vi "Module_ENG_SnakeProcessor.vi"(8 "error in (no error)":errorcluster, 9 "Module ID (-1: Do not Address)":i32=-1, 10 "Wait on Module(s) (\"\": none)":string) -> (0 "error out":errorcluster)   [LabVIEW 2019, in "Module_ENG_SnakeProcessor.lvclass"]
doc: "created using\nJSMA Module Template - ENGINE Class 0.2.1.12\nRob Humfeld - Jet Engineering\nCopyright (c) 2020, Jet Engineering"
uses:
  Module_ENG_SnakeProcessor.lvclass
  <userlib>/Jet Engineering/JET_QSM/Code/Private/JET_QSM - Add State to Front [String API].vi
  Private/Module_ENG_SnakeProcessor_jMsgTxList STYP.ctl
  Private/Module_ENG_SnakeProcessor_jMsgRxList STYP.ctl
  <userlib>/Jet Engineering/JET_QSM/Code/Private/JET_QSM_InvalidOption STYP.ctl
  <userlib>/Jet Engineering/JET_QSM/Code/Private/JET_QSM - Add State [String API].vi
  Private/Module_ENG_SnakeProcessor_EngineStatus STYP.ctl
  Private/Module_ENG_SnakeProcessor_LocalData STYP.ctl
  <userlib>/Jet Engineering/JSMA/Libraries/jMsg_CORE/jMsg_JSMA_ModuleOnline/jMsg_JSMA_ModuleOnline.lvclass
  <userlib>/Jet Engineering/JSMA/Libraries/jMsg_CORE/jMsg_JSMA_ApplicationShutdown/jMsg_JSMA_ApplicationShutdown.lvclass
  <userlib>/Jet Engineering/JSMA/Libraries/jModule Class/jModule.lvclass
  Shared/TCP/jMsgs/jMsg_TCPMessage_Receive/jMsg_TCPMessage_Receive.lvclass
  <userlib>/Jet Engineering/JSMA/Libraries/jMsg Class/jMsg.lvclass
  Shared/TCP/jMsgs/jMsg_TCPMessage_Send/jMsg_TCPMessage_Send.lvclass
  Shared/Board/Board.lvclass
  Shared/jMsgs/jMsg_SnakeProcessor_RemovePlayer/jMsg_SnakeProcessor_RemovePlayer.lvclass
  Shared/jMsgs/jMsg_SnakeProcessor_AddPlayer/jMsg_SnakeProcessor_AddPlayer.lvclass
  Shared/jMsgs/jMsg_SnakeProcessor_ConfigureBoard/jMsg_SnakeProcessor_ConfigureBoard.lvclass
  Shared/jMsgs/jMsg_SnakeProcessor_PauseGame/jMsg_SnakeProcessor_PauseGame.lvclass
  Shared/jMsgs/jMsg_SnakeProcessor_StartGame/jMsg_SnakeProcessor_StartGame.lvclass
  Shared/jMsgs/jMsg_SnakeProcessor_StopGame/jMsg_SnakeProcessor_StopGame.lvclass
  Shared/Player/Player.lvclass
  C:/Program Files/National Instruments/LabVIEW 2019/user.lib/Jet Engineering/JSMA/Libraries/jModule Class/jModule.lvclass
  Shared/jMsgs/jMsg_SnakeProcessor_PlayerUpdate/jMsg_SnakeProcessor_PlayerUpdate.lvclass
  Shared/jMsgs/jMsg_SnakeProcessor_PlayerDeath/jMsg_SnakeProcessor_PlayerDeath.lvclass
  <userlib>/Jet Engineering/JSMA/Libraries/jModule Class/Typedefs/jModule_TimerType STYP.ctl
  <userlib>/Jet Engineering/JSMA/Libraries/jModule Class/Typedefs/jModule_TimerConfig STYP.ctl
panel:
  out "Timer Configuration":T1 {"Expiration Time" format="%<%.3X>T"}
  out "jModule Name":string
  out "iter":i32
  out "Latency, sec.":dbl
  out "RxTime":timestamp format="%<%H:%M:%S%3u>T"
  out "Last Rx Message":string
  out "Recent states before Error (with tick counts)":string
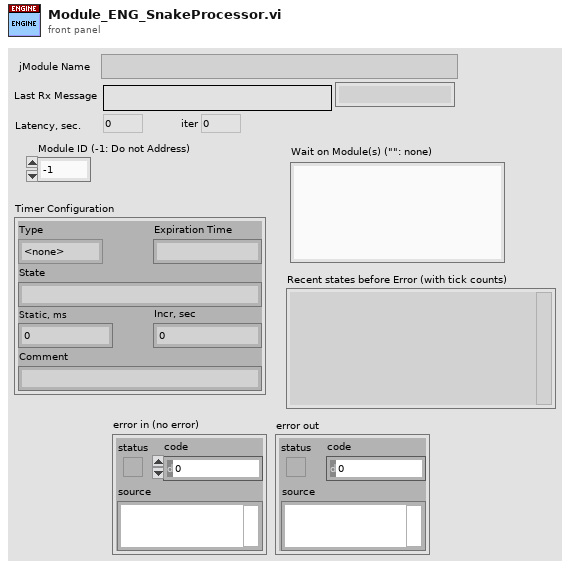
[diagram p1: front panel]
types:
  T1 = typedef "JSMA API.lvlib/jModule.lvclass/jModule_TimerConfig STYP.ctl" = cluster{"Type":T2, "Expiration Time":timestamp, "State":string, "Static, ms":i32, "Incr, sec":dbl, "Comment":string}
  T2 = typedef "JSMA API.lvlib/jModule.lvclass/jModule_TimerType STYP.ctl" = enum16{"<none>", "Static", "Countdown", "Periodic"}
  T3 = typedef "JET_QSM_InvalidOption STYP.ctl" = enum16{"Ignore", "Dialog", "Error"}
  T4 = typedef "Module_ENG_SnakeProcessor.lvclass/Module_ENG_SnakeProcessor_LocalData STYP.ctl" = cluster{"VI":cluster{"error":errorcluster, "isExiting?":bool}, "EngineStatus":T5}
  T5 = typedef "Module_ENG_SnakeProcessor.lvclass/Module_ENG_SnakeProcessor_EngineStatus STYP.ctl" = cluster{"Board":refnum<class "Board.lvclass">, "Tick":u64, "Game Settings":cluster{"Tick Rate (ms)":u32, "Food Probability (%)":dbl, "Height":i32, "Width":i32}, "Game Started?":bool}
  T6 = typedef "Module_ENG_SnakeProcessor.lvclass/Module_ENG_SnakeProcessor_jMsgRxList STYP.ctl" = cluster{"<placeholder>":refnum<class "jMsg_JSMA_ApplicationShutdown.lvclass">, "jMsg_TCPMessage_Receive":refnum<class "jMsg_TCPMessage_Receive.lvclass">, "jMsg_SnakeProcessor_ConfigureBoard":refnum<class "jMsg_SnakeProcessor_ConfigureBoard.lvclass">, "jMsg_SnakeProcessor_AddPlayer":refnum<class "jMsg_SnakeProcessor_AddPlayer.lvclass">, "jMsg_SnakeProcessor_RemovePlayer":refnum<class "jMsg_SnakeProcessor_RemovePlayer.lvclass">, "jMsg_SnakeProcessor_StartGame":refnum<class "jMsg_SnakeProcessor_StartGame.lvclass">, "jMsg_SnakeProcessor_PauseGame":refnum<class "jMsg_SnakeProcessor_PauseGame.lvclass">, "jMsg_SnakeProcessor_StopGame":refnum<class "jMsg_SnakeProcessor_StopGame.lvclass">}
  T7 = typedef "Module_ENG_SnakeProcessor.lvclass/Module_ENG_SnakeProcessor_jMsgTxList STYP.ctl" = cluster{"<placeholder>":refnum<class "jMsg_JSMA_ModuleOnline.lvclass">, "jMsg_TCPMessage_Send":refnum<class "jMsg_TCPMessage_Send.lvclass">, "jMsg_SnakeProcessor_PlayerDeath":refnum<class "jMsg_SnakeProcessor_PlayerDeath.lvclass">, "jMsg_SnakeProcessor_PlayerUpdate":refnum<class "jMsg_SnakeProcessor_PlayerUpdate.lvclass">}
  T8 = typedef "JET_QSM_Refnum STYP.ctl" = cluster{"state":cluster{"queue":refnum<queue>, "idle":string, "error":string, "STOP":string}, "debug":cluster{"enabled?":bool, "queue":refnum<queue>}, "Invalid.option":T3, "QSM.Name":string}
  T9 = typedef "JET_QSM_Element STYP.ctl" = cluster{"state":string, "data":variant, "comment":string}
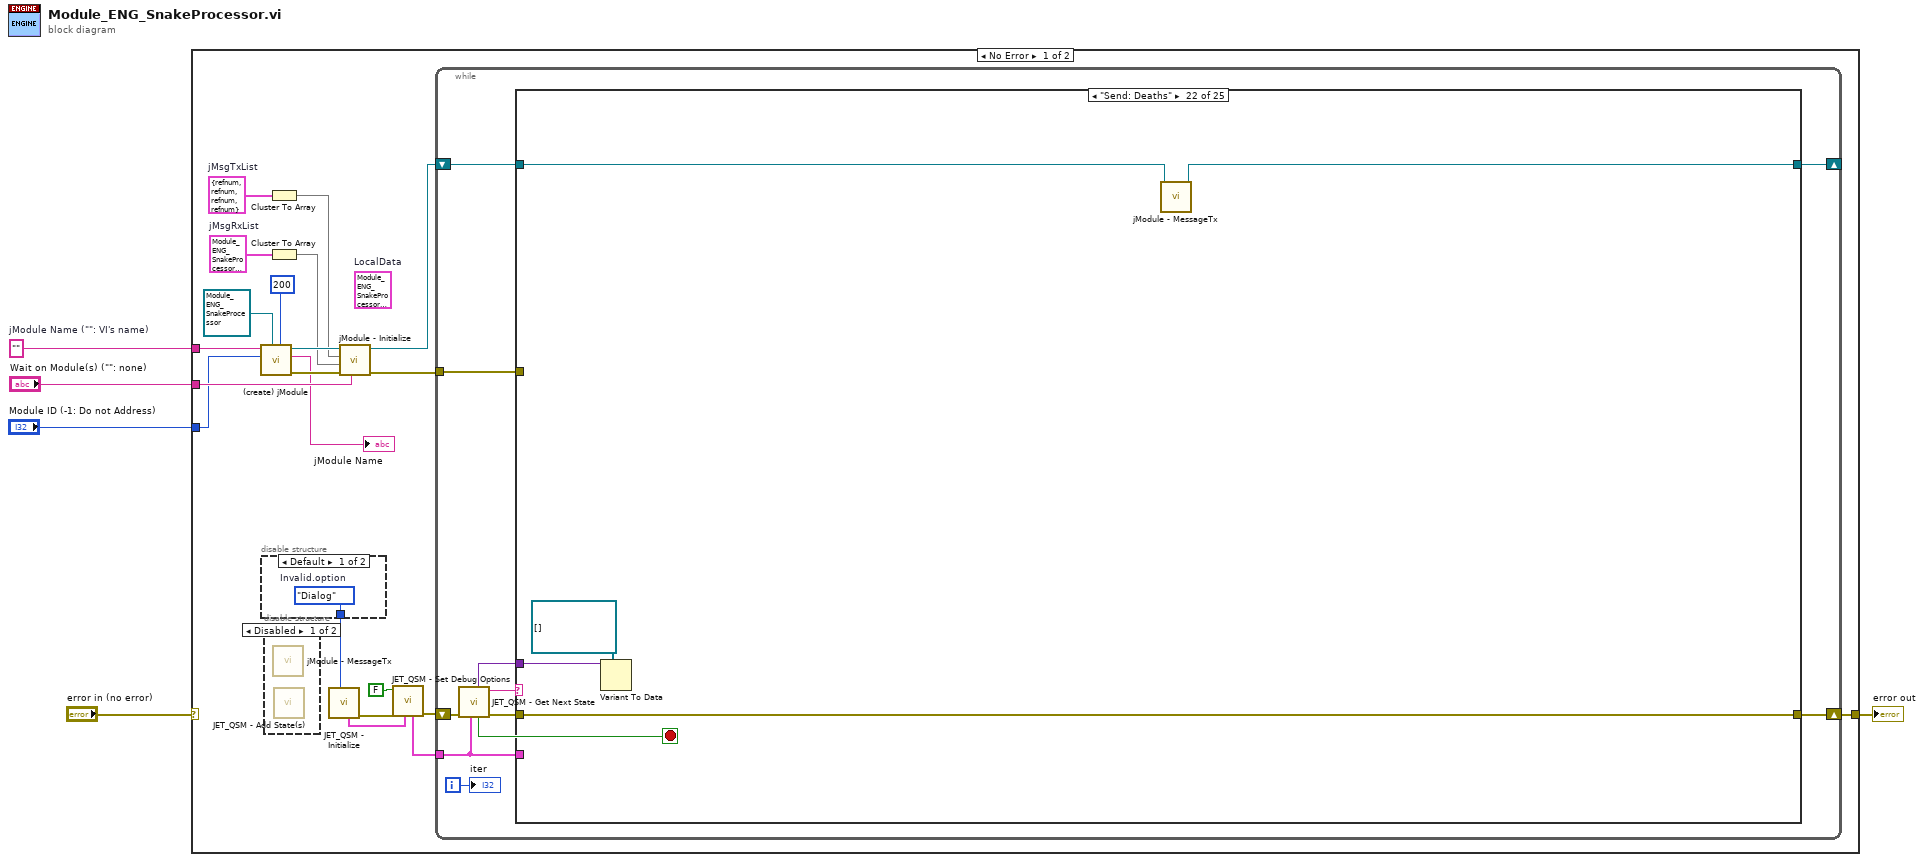
[diagram p0: block diagram]
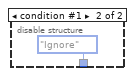
[diagram p3: hidden frame]
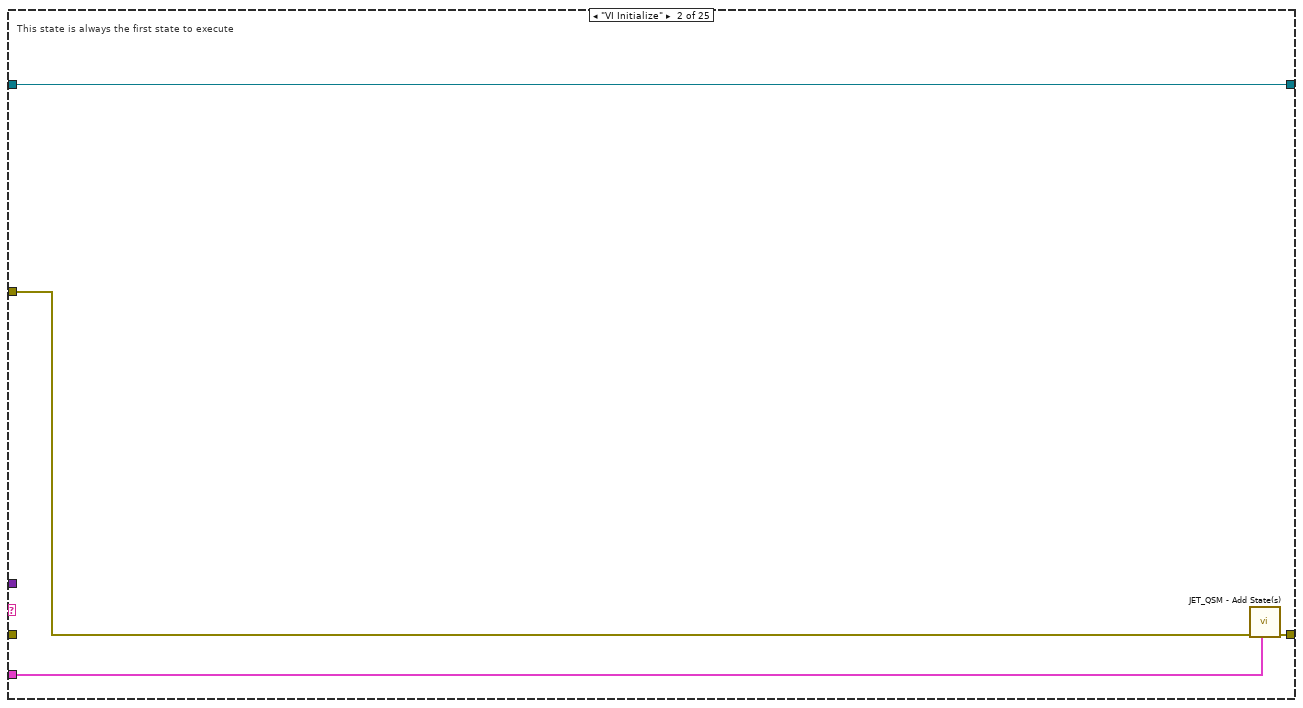
[diagram p5: hidden frame]
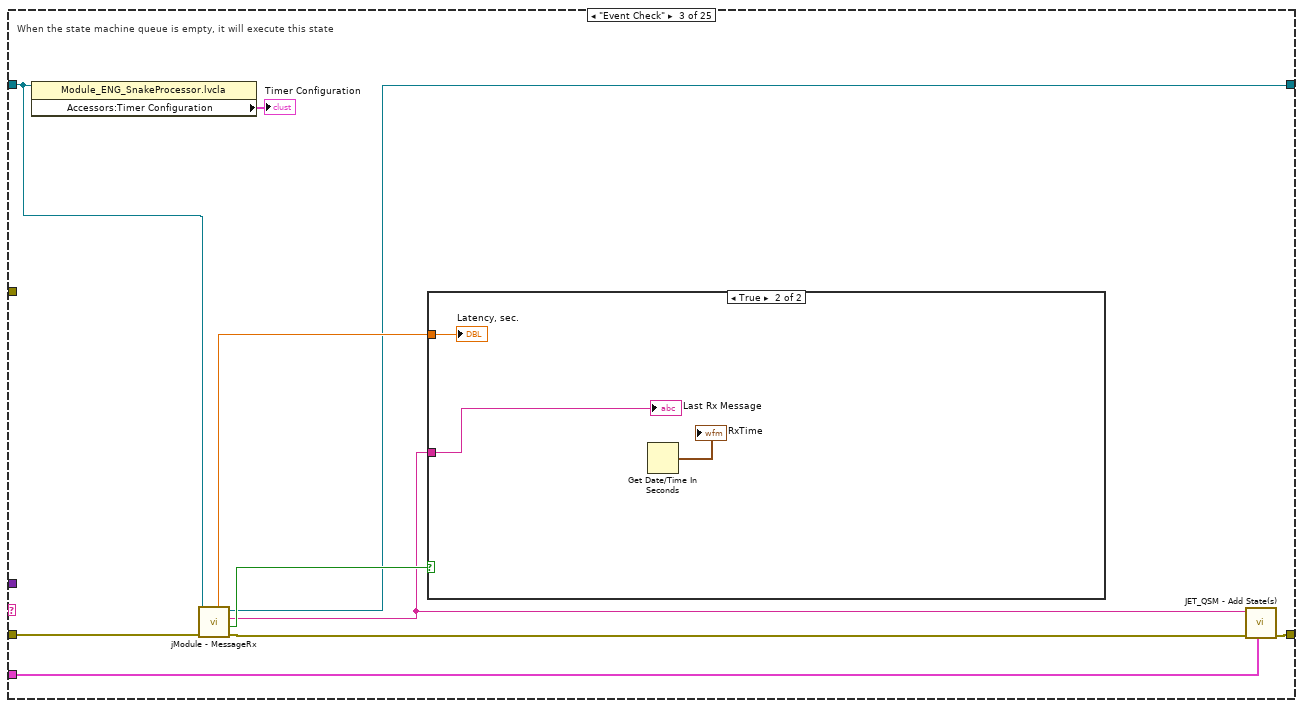
[diagram p6: hidden frame]
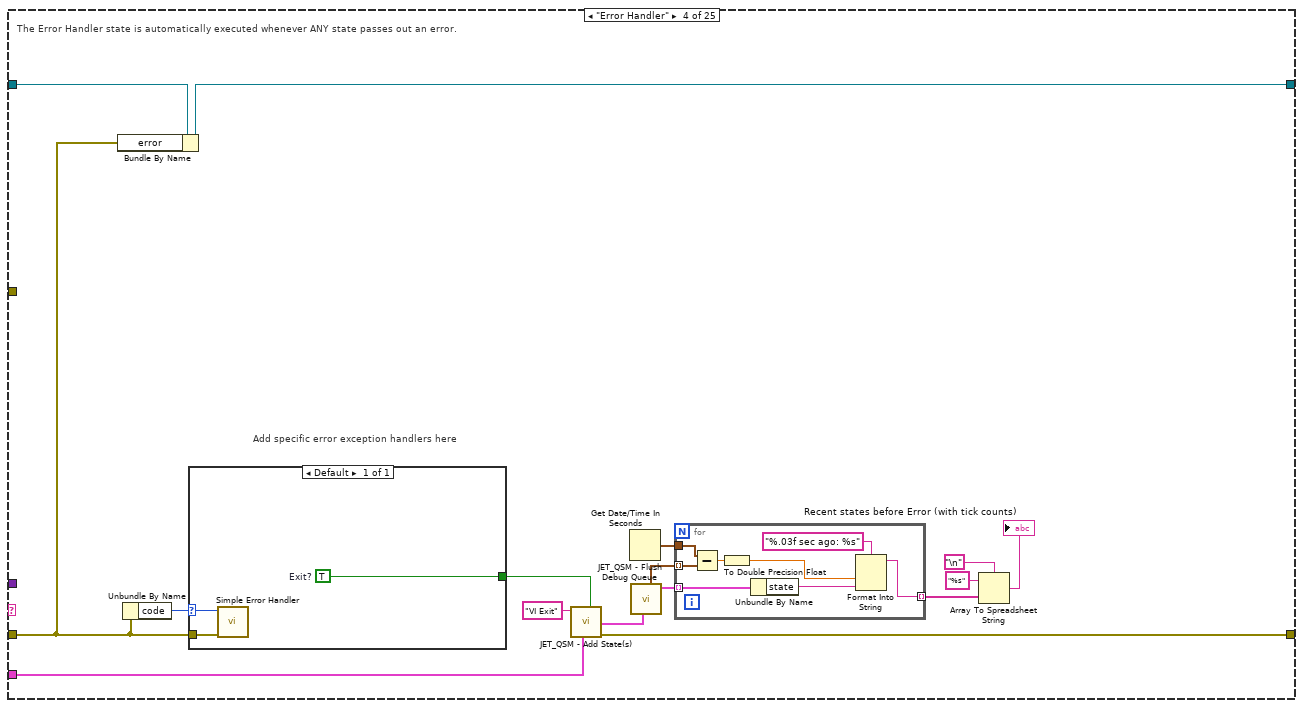
[diagram p8: hidden frame]
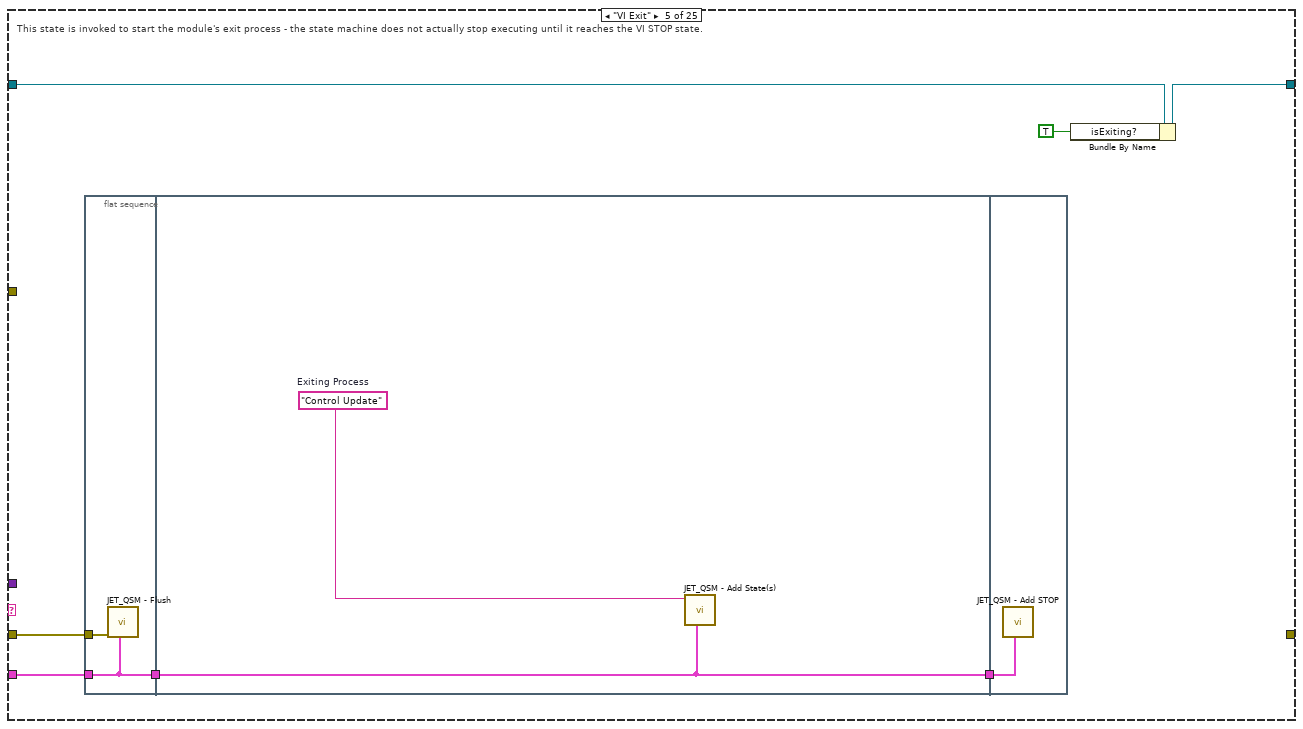
[diagram p9: hidden frame]
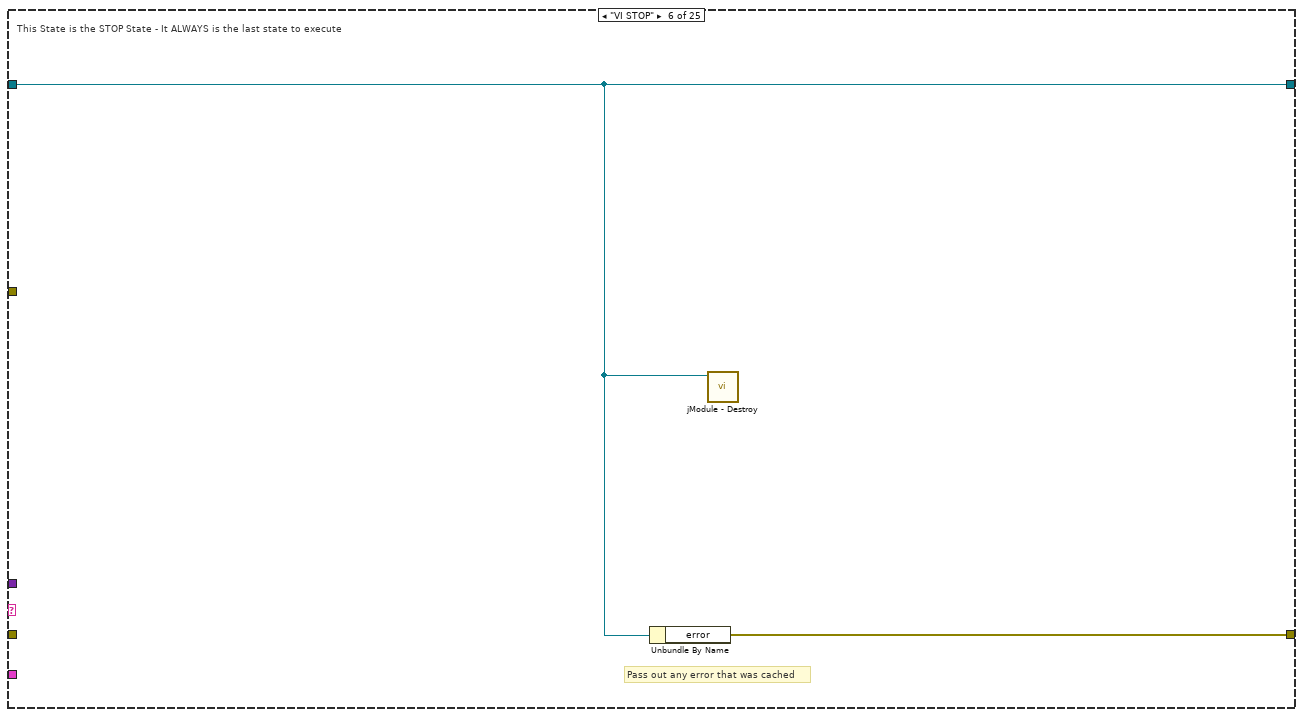
[diagram p10: hidden frame]
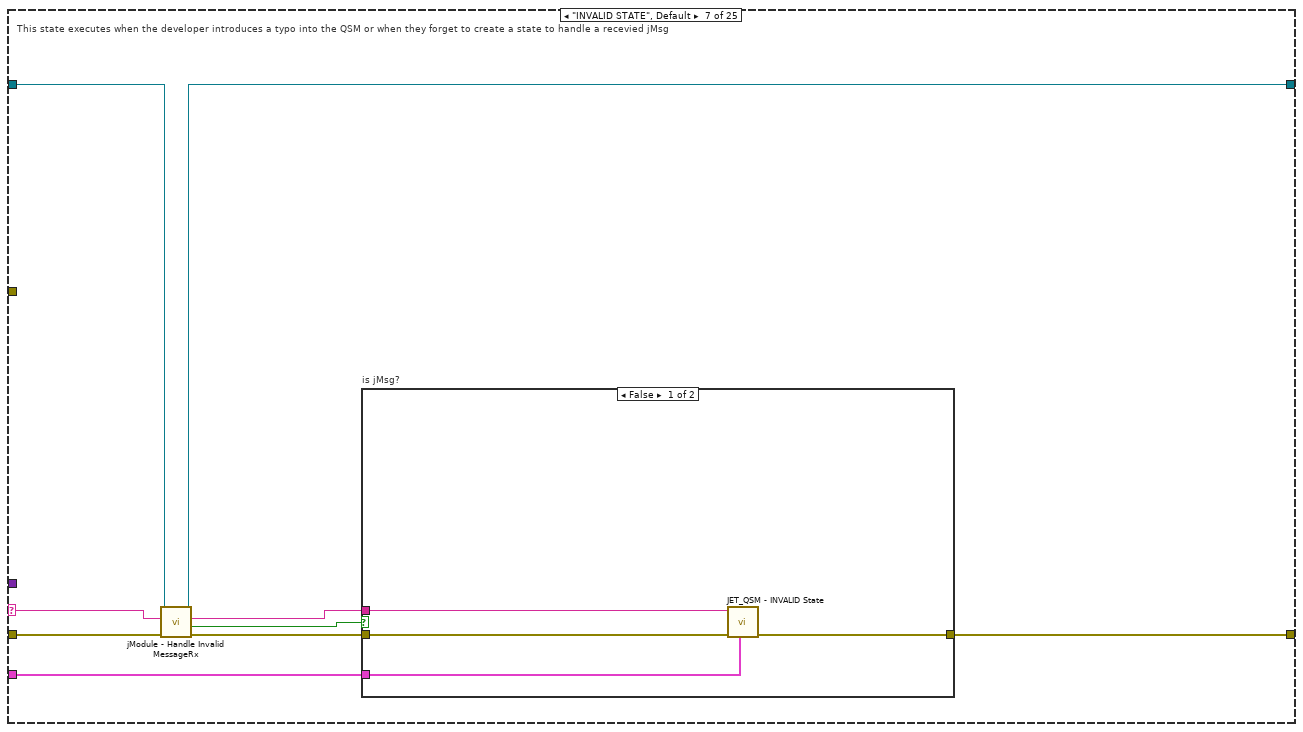
[diagram p11: hidden frame]
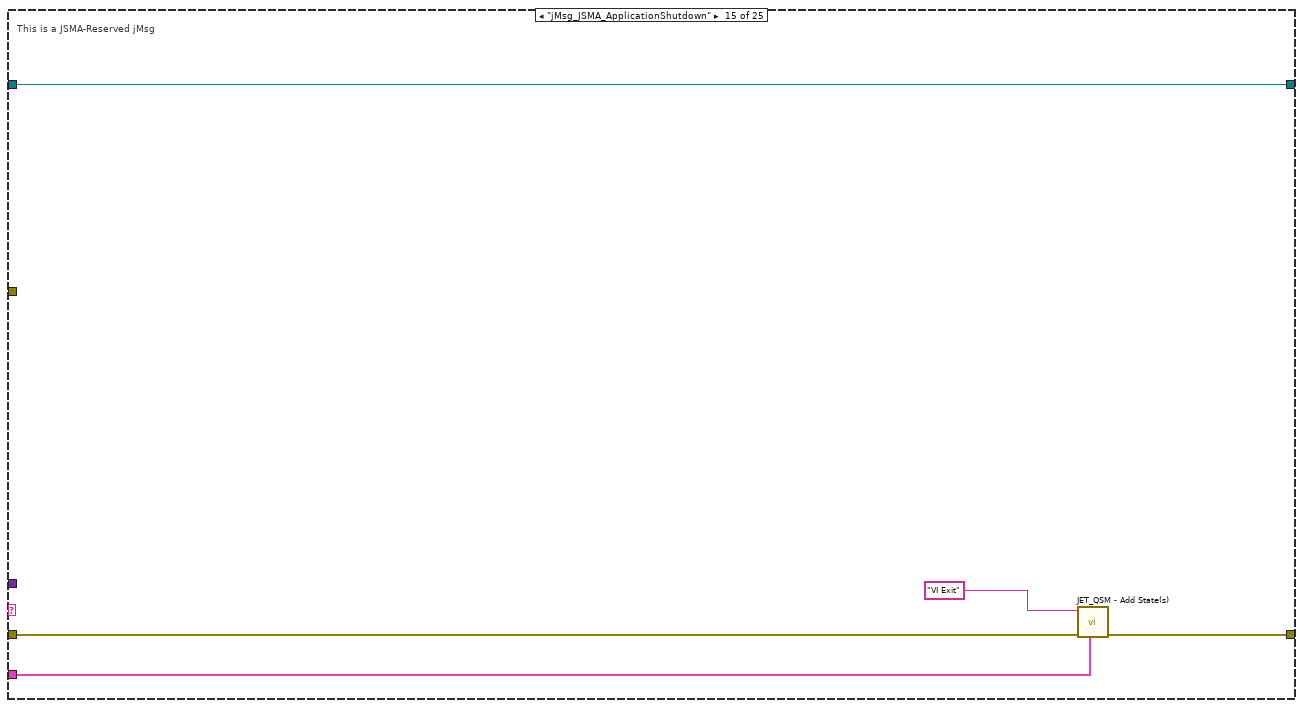
[diagram p20: hidden frame]
diagram:
  w3 = ""  # jModule Name ("": VI's name)
  n1 = case shown="No Error" "error in (no error)" {
    selector: "error in (no error)" -> [_ w191]
    tunnel: [w9 w191] -> w5
    tunnel: "Wait on Module(s) (\"\": none)" -> [w17 _]
    tunnel: w3 -> [w16 _]
    tunnel: "Module ID (-1: Do not Address)" -> [w8 _]
    frame No Error {
      (unwired) T4 {"VI"={"error"={"status"=FALSE, "code"=0, "source"=""}, "isExiting?"=FALSE}, "EngineStatus"={"Board"=refnum, "Tick"=0, "Game Settings"={"Tick Rate (ms)"=0, "Food Probability (%)"=0.0, "Height"=0, "Width"=0}, "Game Started?"=FALSE}}  # LocalData
      w14 = T6 {"<placeholder>"=refnum, "jMsg_TCPMessage_Receive"=refnum, "jMsg_SnakeProcessor_ConfigureBoard"=refnum, "jMsg_SnakeProcessor_AddPlayer"=refnum, "jMsg_SnakeProcessor_RemovePlayer"=refnum, "jMsg_SnakeProcessor_StartGame"=refnum, "jMsg_SnakeProcessor_PauseGame"=refnum, "jMsg_SnakeProcessor_StopGame"=refnum}  # jMsgRxList
      w15 = T7 {"<placeholder>"=refnum, "jMsg_TCPMessage_Send"=refnum, "jMsg_SnakeProcessor_PlayerDeath"=refnum, "jMsg_SnakeProcessor_PlayerUpdate"=refnum}  # jMsgTxList
      n2 = call <userlib>:"(create) jModule.vi"("Max Queue size (50)"=200, "jModule Child class"=refnum<class "Module_ENG_SnakeProcessor.lvclass"> refnum ("jModule Template_ENGINEClass.lvclass"), "Module ID (-1: Do Not Address)"=w8, "jModule Name (\"\": use calling VI's name)"=w16) -> ("error out"=w19:errorcluster, "jModule Name"=→"jModule Name":string, "jModule"=w22:refnum<class "Module_ENG_SnakeProcessor.lvclass">)  [unwired: 4 in, 1 out]
      n3 = disable-structure shown="Default" {
        disable-tunnel: [w27 JET_QSM_InvalidOption_STYP."Ignore" ("Invalid.option (Dialog)")] -> w18
        frame condition #0 (active) {
          w27 = JET_QSM_InvalidOption_STYP."Dialog"  # Invalid.option
        }
        frame condition #1 {
        }
      }
      n4 = disable-structure shown="Disabled" {
        frame Disabled {
          n5 = call <userlib>:"jModule - MessageTx.vi"() -> ()  [unwired: 8 in, 4 out]
          n6 = call-poly <userlib>:"JET_QSM - Add State(s).vi"() -> ()  [unwired: 11 in, 1 out]
        }
        frame Enabled {
        }
      }
      n7 = Cluster To Array(cluster=w15) -> (array=w21:refnum<class "jMsg.lvclass">[])
      n8 = Cluster To Array(cluster=w14) -> (array=w20:refnum<class "jMsg.lvclass">[])
      n9 = call <userlib>:"JET_QSM - Initialize.vi"("invalid state action (Dialog)"=w18) -> ("error out"=w23:errorcluster, "Jet_QSM refnum"=w25:T8)  [unwired: 9 in]
      n10 = call-dynamic "jModule - Initialize.vi"("Wait on Module(s) (\"\": none)"=w17, "error in (no error)"=w19, "jMsgRxList"=w20, "jMsgTxList"=w21, "jModule"=w22) -> ("error out"=w11:errorcluster, "jModule"=w10:refnum<class "Module_ENG_SnakeProcessor.lvclass">)  [unwired: 5 in]
      n11 = call <userlib>:"JET_QSM - Set Debug Options.vi"("Jet_QSM refnum"=w25, "error in (no error)"=w23, "debug.enabled? (F)"=FALSE) -> ("error out"=w12:errorcluster, "Jet_QSM ref"=w24:T8)  [unwired: 7 in]
      n12 = while {
        tunnel: w24 -> [w30]
        shift-right: [w34] -> _
        shift-left: w10 -> [w35]
        shift-right: [w33] -> w9
        shift-left: w12 -> [w39]
        tunnel: w11 -> [w31]
        i -> [w32]
        stop <- w36 stop-if-true
        n13 = call <userlib>:"JET_QSM - Get Next State.vi"("Jet_QSM refnum"=w30, "error in (no error)"=w39) -> ("error out"=w38:errorcluster, "state"=w37:string, "Stop Loop?"=w36:bool, "state data"=w29:variant)  [unwired: 5 in, 1 out]
        n14 = case shown="\"Send: Deaths\"" w37 {
          selector: w37 -> [_ _ _ _ _ _ w103 _ _ _ _ _ _ _ _ _ _ _ _ _ _ _ _ _ _]
          tunnel: w38 -> [w40 _ w53 w63 w91 _ w104 w113 w115 w117 w119 w121 w123 w125 w127 w132 w142 w149 w154 w160 w169 w181 w182 w184 w189]
          tunnel: w35 -> [w41 w43 w49 w60 w86 w98 w100 w114 w116 w118 w120 w122 w124 w126 w128 w133 w136 w144 w152 w162 w167 w177 w183 w185 w190]
          tunnel: [w41 w43 w47 w59 w85 w98 w99 w114 w116 w118 w120 w122 w124 w126 w128 w133 w140 w148 w151 w163 w170 w178 w183 w185 w190] -> w34
          tunnel: [w40 w45 w54 w66 _ w97 w102 w113 w115 w117 w119 w121 w123 w125 w130 w132 w142 w149 w154 w161 w168 w181 w182 w187 w189] -> w33
          tunnel: w31 -> [_ w42 _ _ _ _ _ _ _ _ _ _ _ _ _ _ _ _ _ _ _ _ _ _ _]
          tunnel: w30 -> [_ w44 w55 w65 w90 _ w101 _ _ _ _ _ _ _ w131 _ _ _ _ w159 _ _ _ w188 _]
          tunnel: w29 -> [_ _ _ _ _ _ _ _ _ _ _ _ _ _ _ _ _ _ _ _ _ w180 _ _ _]
          frame "------ Standard States ------" {
            # "Standard States are required states for a JET_QSM State Machine\n\nTheir names may be changed; use the Initialize function to specify the new names"
            # "This is a section header; the state is never expected to execute"
          }
          frame "VI Initialize" {
            # "This state is always the first state to execute"
            n15 = call-poly <userlib>:"JET_QSM - Add State(s).vi"("Jet_QSM refnum"=w44, "error in (no error)"=w42) -> ("error out"=w45:errorcluster)  [unwired: 9 in]
          }
          frame "Event Check" {
            # "When the state machine queue is empty, it will execute this state"
            n16 = property class="Module_ENG_SnakeProcessor.lvcla"(reference=w49) -> ("Accessors:Timer Configuration"=→"Timer Configuration":T1)  [unwired: 1 in, 2 out]
            n17 = call-dynamic "jModule - MessageRx.vi"("error in (no error)"=w53, "jModule"=w49) -> ("error out"=w48:errorcluster, "MsgRx?"=w52:bool, "QSMState"=w50:string, "jModule"=w47:refnum<class "Module_ENG_SnakeProcessor.lvclass">, "Latency, sec."=w51:dbl)  [unwired: 4 in, 1 out]
            n18 = case shown="True" w52 {
              tunnel: w50 -> [_ w57]
              tunnel: w51 -> [_ w58]
              frame False {
              }
              frame True {
                n19 = Get Date/Time In Seconds() -> (seconds since 1Jan1904=→"RxTime":timestamp)
                "Last Rx Message" <- w57
                "Latency, sec." <- w58
              }
            }
            n20 = call-poly <userlib>:"JET_QSM - Add State(s).vi"("Jet_QSM refnum"=w55, "error in (no error)"=w48, "state(s)"=w50) -> ("error out"=w54:errorcluster)  [unwired: 8 in]
          }
          frame "Error Handler" {
            # "Add specific error exception handlers here"
            # "The Error Handler state is automatically executed whenever ANY state passes out an error."
            n21 = Bundle By Name(cluster=w60, "error"=w63) -> (w59:refnum<class "Module_ENG_SnakeProcessor.lvclass">)
            n22 = Unbundle By Name(w63) -> ("code"=w61:i32)
            n23 = case shown="Default" w61 {
              selector: w61 -> [w75]
              tunnel: [w76] -> w62
              tunnel: w63 -> [w74]
              frame Default {
                w76 = TRUE  # Exit?
                n24 = call <vilib>:"Simple Error Handler.vi"("error code (no error:0)"=w75, "error in (no error)"=w74) -> ()  [unwired: 3 in, 5 out]
              }
            }
            n25 = call-poly <userlib>:"JET_QSM - Add State(s).vi"("act? (T)"=w62, "Jet_QSM refnum"=w65, "state(s)"="VI Exit") -> ("error out"=w66:errorcluster)  [unwired: 8 in]
            n26 = Get Date/Time In Seconds() -> (seconds since 1Jan1904=w69:timestamp)
            n27 = call <userlib>:"JET_QSM - Flush Debug Queue.vi"("Jet_QSM refnum"=w65) -> ("QSM Elements"=w67:T9[], "Timestamps"=w68:timestamp[])  [unwired: 8 in, 1 out]
            n28 = for {
              tunnel: w67 -> [w84] mode=indexing
              tunnel: [w82] -> w71 mode=indexing
              tunnel: w69 -> [w79]
              tunnel: w68 -> [w80] mode=indexing
              n29 = Subtract(x=w79, y=w80) -> (x-y=w78:dbl)
              n30 = To Double Precision Float(number=w78) -> (double precision float=w77:dbl)
              n31 = Unbundle By Name(w84) -> ("state"=w83:string)
              n32 = Format Into String(format string="%.03f sec ago: %s", w77, w83) -> (resulting string=w82:string)  [unwired: 2 in, 1 out]
            }
            n33 = Array To Spreadsheet String(delimiter (Tab)="\n", array=w71, 3:"%s" ("format string")) -> (spreadsheet string=→"Recent states before Error (with tick counts)":string)
          }
          frame "VI Exit" {
            # "This state is invoked to start the module's exit process - the state machine does not actually stop executing until it reaches the VI STOP state."
            n34 = flat-sequence {
              tunnel: w91 -> [w93]
              tunnel: w90 -> [w92]
              tunnel: [w92] -> w89
              tunnel: w89 -> [w95]
              tunnel: [w95] -> w88
              tunnel: w88 -> [w96]
              frame #0 {
                n35 = call <userlib>:"JET_QSM - Flush.vi"("Jet_QSM ref"=w92, "error in (no error)"=w93) -> ()  [unwired: 8 in, 2 out]
              }
              frame #1 {
                w94 = "Control Update"  # Exiting Process
                n36 = call-poly <userlib>:"JET_QSM - Add State(s).vi"("Jet_QSM refnum"=w95, "state(s)"=w94) -> ()  [unwired: 9 in, 1 out]
              }
              frame #2 {
                n37 = call <userlib>:"JET_QSM - Add STOP.vi"("Jet_QSM refnum"=w96) -> ()  [unwired: 10 in, 1 out]
              }
            }
            n38 = Bundle By Name(cluster=w86, "isExiting?"=TRUE ("VI.isExiting?")) -> (w85:refnum<class "Module_ENG_SnakeProcessor.lvclass">)
          }
          frame "VI STOP" {
            # "Pass out any error that was cached"
            # "This State is the STOP State - It ALWAYS is the last state to execute"
            n39 = Unbundle By Name(w98) -> ("error"=w97:errorcluster)
            n40 = call-dynamic "jModule - Destroy.vi"("jModule"=w98) -> ()  [unwired: 10 in, 1 out]
          }
          frame "INVALID STATE", Default {
            # "This state executes when the developer introduces a typo into the QSM or when they forget to create a state to handle a recevied jMsg"
            n41 = call-dynamic "jModule - Handle Invalid MessageRx.vi"("error in (no error)"=w104, "Invalid State"=w103, "jModule"=w100) -> ("error out"=w107:errorcluster, "is jMsg State?"=w105:bool, "Invalid State"=w106:string, "jModule"=w99:refnum<class "Module_ENG_SnakeProcessor.lvclass">)  [unwired: 5 in]
            n42 = case "is jMsg?" shown="False" w105 {
              tunnel: w101 -> [w109 _]
              tunnel: [w108 w112] -> w102
              tunnel: w107 -> [w110 w112]
              tunnel: w106 -> [w111 _]
              frame False {
                n43 = call <userlib>:"JET_QSM - INVALID State.vi"("Jet_QSM refnum"=w109, "error in (no error)"=w110, "state"=w111) -> ("error out"=w108:errorcluster)  [unwired: 8 in]
              }
              frame True {
              }
            }
          }
          frame "------ jMsg  ------" {
            # "This is a section header; the state is never expected to execute"
          }
          frame "jMsg_SnakeProcessor_ConfigureBoard" {
          }
          frame "jMsg_SnakeProcessor_AddPlayer" {
          }
          frame "jMsg_SnakeProcessor_RemovePlayer" {
          }
          frame "jMsg_SnakeProcessor_StartGame" {
          }
          frame "jMsg_SnakeProcessor_PauseGame" {
          }
          frame "jMsg_SnakeProcessor_StopGame" {
          }
          frame "jMsg_JSMA_ApplicationShutdown" {
            # "This is a JSMA-Reserved jMsg"
            n44 = call-poly <userlib>:"JET_QSM - Add State(s).vi"("Jet_QSM refnum"=w131, "error in (no error)"=w127, "state(s)"="VI Exit") -> ("error out"=w130:errorcluster)  [unwired: 8 in]
          }
          frame "------ Actions  ------" {
            # "This is a section header; the state is never expected to execute"
          }
          frame "Game: Initialize" {
            n45 = Unbundle By Name(w136) -> ("Height"=w135:i32, "Width"=w134:i32)
            n46 = call "create Board.vi"("Height"=w135, "Width"=w134, "Players"=refnum<class "Player.lvclass">[] []) -> ("Board out"=w137:refnum<class "Board.lvclass">)  [unwired: 7 in, 1 out]
            n47 = Bundle By Name(cluster=w136, "Board"=w137, "Tick"=u64 0 ("My.EngineStatus.Tick"), "Game Started?"=FALSE ("My.EngineStatus.Game Started?")) -> (w140:refnum<class "Module_ENG_SnakeProcessor.lvclass">)
          }
          frame "Game: Start" {
            n48 = Unbundle By Name(w144) -> ("Tick Rate (ms)"=w143:u32)
            n49 = call <userlib>:"jModule - Set Periodic Timer.vi"("Go to State Periodically (\"\": no change)"="Game: Tick" ("Go to State Periodically (\"\": no change)"), "Timing Period, ms"=w143, "jModule"=w144) -> ("jModule"=w146:refnum<class "Module_ENG_SnakeProcessor.lvclass">)  [unwired: 7 in, 1 out]
            n50 = Bundle By Name(cluster=w146, "Game Started?"=TRUE ("My.EngineStatus.Game Started?")) -> (w148:refnum<class "Module_ENG_SnakeProcessor.lvclass">)
          }
          frame "Game: Stop" {
            n51 = call <userlib>:"jModule - Set Static Timer.vi"("jModule"=w152) -> ("jModule"=w153:refnum<class "Module_ENG_SnakeProcessor.lvclass">)  [unwired: 9 in, 1 out]
            n52 = Bundle By Name(cluster=w153, "Game Started?"=FALSE ("My.EngineStatus.Game Started?")) -> (w151:refnum<class "Module_ENG_SnakeProcessor.lvclass">)
          }
          frame "Game: Tick" {
            n53 = in-place {
              in-place-border: [w164] -> w157
              n54 = in-place-cluster #1(w162) -> ("Board"=w166:refnum<class "Board.lvclass">)
              n55 = call-dynamic "Board Tick.vi"("Board in"=w166) -> ("Dead Players"=w164:refnum<class "Player.lvclass">[], "Board out"=w165:refnum<class "Board.lvclass">)  [unwired: 8 in, 1 out]
              n56 = in-place-cluster #1("Board"=w165) -> (w163:refnum<class "Module_ENG_SnakeProcessor.lvclass">)
            }
            n57 = Array Size(array=w157) -> (size(s)=w156:i32)
            n58 = Greater Than 0?(x=w156) -> (x > 0?=w155:bool)
            n59 = call-poly <userlib>:"JET_QSM - Add State(s).vi"("act? (T)"=w155, "Jet_QSM refnum"=w159, "error in (no error)"=w160, "state(s) data [ALL states]"=w157, "state(s)"="Send: Deaths") -> ("error out"=w161:errorcluster)  [unwired: 6 in]
          }
          frame "Send: Status Update" {
            # "This is how your engine broadcasts its status to the application"
            n60 = disable-structure shown="Enabled" {
              disable-tunnel: [w173 w176] -> w170
              disable-tunnel: w169 -> [w172 w175]
              disable-tunnel: [w171 w175] -> w168
              disable-tunnel: w167 -> [w174 w176]
              frame Disabled {
                # "Create a jMsg\nfor this"
                n61 = Unbundle By Name(w174) -> ()  [unwired: 1 out]
                n62 = call <userlib>:"jModule - MessageTx.vi"("error in (no error)"=w172, "jModule"=w174) -> ("error out"=w171:errorcluster, "jModule"=w173:refnum<class "Module_ENG_SnakeProcessor.lvclass">)  [unwired: 6 in, 2 out]
              }
              frame Enabled {
              }
            }
          }
          frame "Send: Deaths" {
            n63 = Variant To Data(type=refnum<class "Player.lvclass">[] [], Variant=w180) -> ()  [unwired: 1 in, 2 out]
            n64 = call <userlib>:"jModule - MessageTx.vi"("jModule"=w177) -> ("jModule"=w178:refnum<class "Module_ENG_SnakeProcessor.lvclass">)  [unwired: 7 in, 3 out]
          }
          frame "------ Window and Panel Control ------" {
            # "This is a section header; the state is never expected to execute"
          }
          frame "Control Update" {
            # "Update all control properties values from the status cluster in this state - in this way we can separate the View from the Model and Controller, as well as consolidate/reduce locals and property nodes"
            n65 = call-poly <userlib>:"JET_QSM - Add State(s).vi"("Jet_QSM refnum"=w188, "error in (no error)"=w184, "state(s)"="Indicator Update") -> ("error out"=w187:errorcluster)  [unwired: 8 in]
          }
          frame "Indicator Update" {
            # "Update all indicator properties and values from the status cluster in this state - in this way we can separate the View from the Model and Controller, as well as consolidate/reduce property nodes"
          }
        }
        "iter" <- w32
      }
    }
    frame Error {
    }
  }
  "error out" <- w5
